vi "getPathPrivate.vi"(1 "bentStyleRef":refnum<class "BentStyle.lvclass">, 2 "start":T2 {"height" format="%.2f"; "width" format="%.2f"; "y" format="%.2f"; "x" format="%.2f"}, 3 "end":T2 {"height" format="%.2f"; "width" format="%.2f"; "y" format="%.2f"; "x" format="%.2f"}, 5 "error in (no error)":errorcluster) -> (15 "path":T3[](array[typedef]) {"y" format="%.2f"; "x" format="%.2f"}, 16 "ok":bool, 17 "startDirection":T1, 18 "endDirection":T1, 19 "error out":errorcluster)   [LabVIEW 2016, in "BentStyle.lvclass"]
doc: "/**\n Gets the points at which a line joining two rectangles\n is bent according to a bent style.\n @param start the starting rectangle\n @param end the ending rectangle\n @return an array list of points at which to bend the\n segmented line joining the two rectangles\n */\n private static ArrayList getPath(BentStyle bent, \n Rectangle2D s, Rectangle2D e)"
uses:
  <resource>/Framework/Providers/Open_GDS/UML/BentStyle_class/BentStyle.lvclass
  <resource>/Framework/Providers/Open_GDS/UML/General/Point/Point Point2D.ctl
  <resource>/Framework/Providers/Open_GDS/UML/General/Rectangle/Rectangle Rectangle2D.ctl
  <resource>/Framework/Providers/Open_GDS/UML/Direction_class/DirectionTypes.ctl
  <resource>/Framework/Providers/Open_GDS/UML/BentStyle_class/BentStyle.lvclass/BentStyle.ctl
  <resource>/Framework/Providers/Open_GDS/UML/Direction_class/Direction.lvclass
panel:
  # "PRIVATE STATIC getPath (BentStyle,Rect,Rect)"
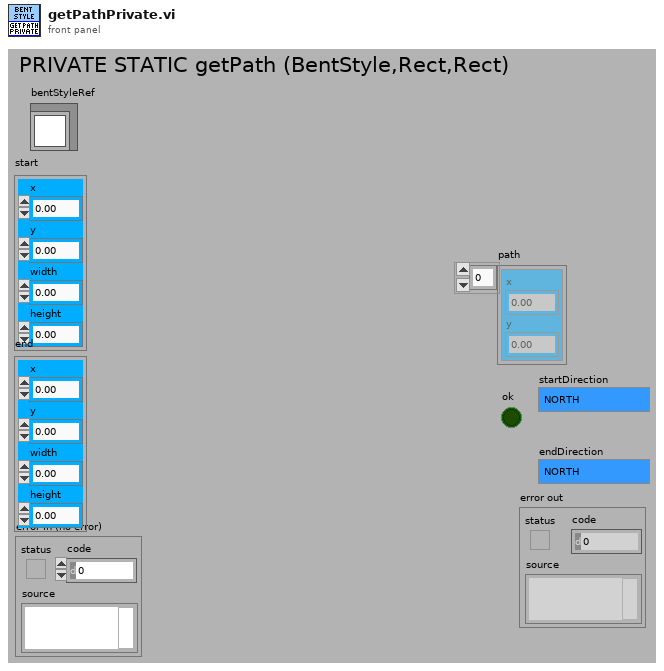
[diagram p1: front panel]
types:
  T1 = typedef "Direction.lvclass/DirectionTypes.ctl" = enum16{"NORTH", "SOUTH", "EAST", "WEST"}
  T2 = typedef "Rectangle Rectangle2D.ctl" = cluster{"x":dbl, "y":dbl, "width":dbl, "height":dbl}
  T3 = typedef "Point Point2D.ctl" = cluster{"x":dbl, "y":dbl}
  T4 = typedef "BentStyle.lvclass/BentStyleType.ctl" = enum16{"STRAIGHT", "HV", "VH", "HVH", "VHV", "ARC"}
  T5 = cluster{"point2D":T3, "point2D":T3, "distance":dbl, i32, i32}
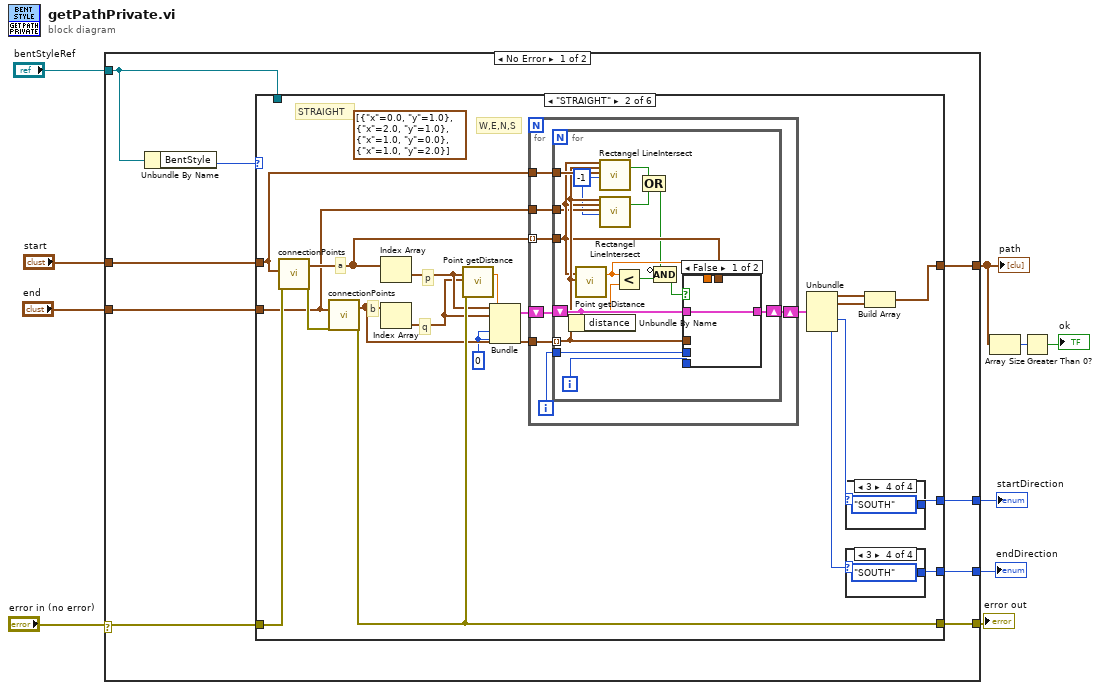
[diagram p0: block diagram]
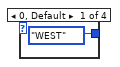
[diagram p3: hidden frame]
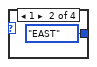
[diagram p4: hidden frame]
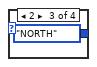
[diagram p5: hidden frame]
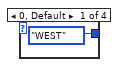
[diagram p6: hidden frame]
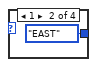
[diagram p7: hidden frame]
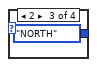
[diagram p8: hidden frame]
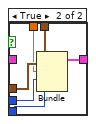
[diagram p9: hidden frame]
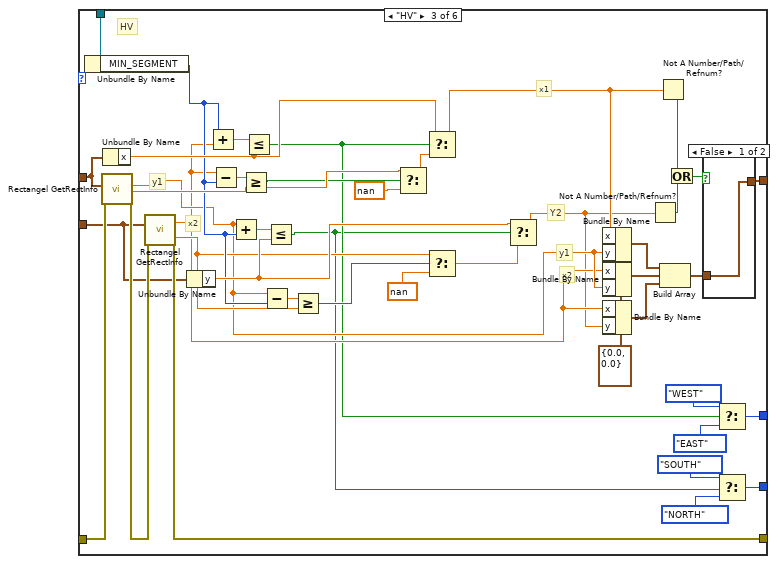
[diagram p10: hidden frame]
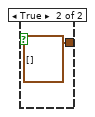
[diagram p11: hidden frame]
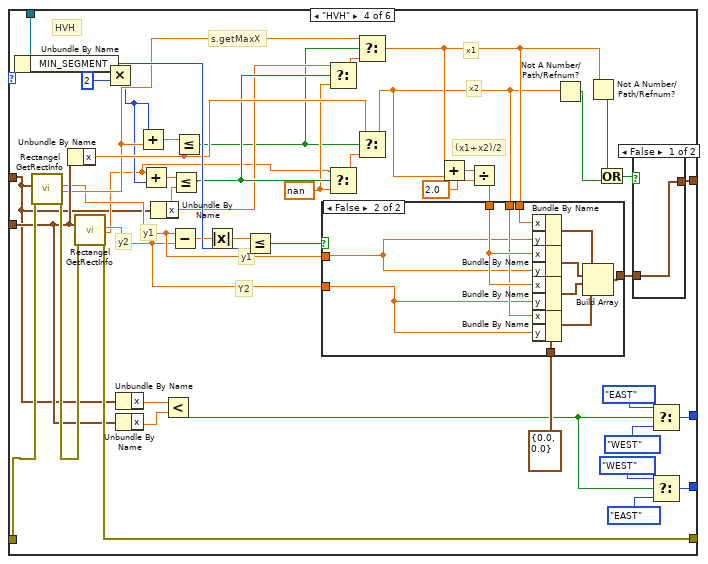
[diagram p12: hidden frame]
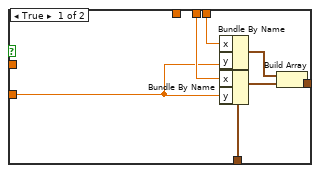
[diagram p13: hidden frame]
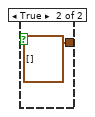
[diagram p14: hidden frame]
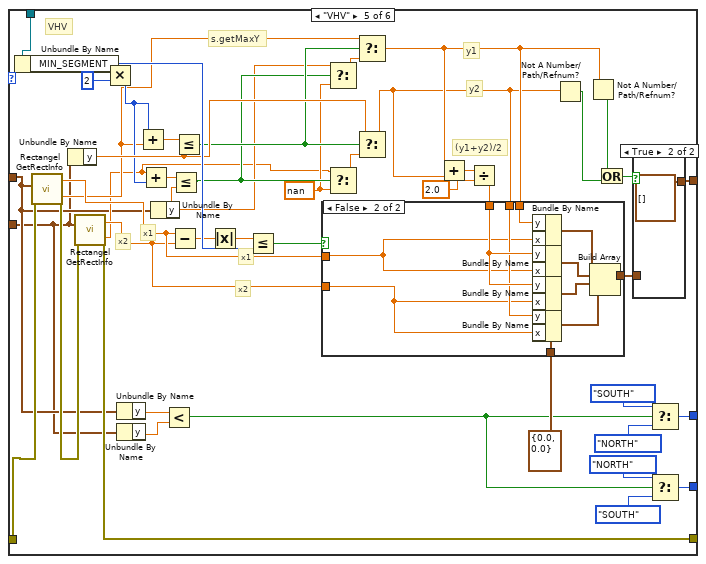
[diagram p15: hidden frame]
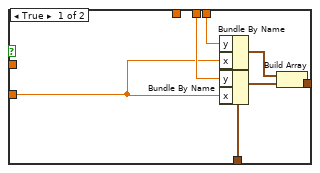
[diagram p16: hidden frame]
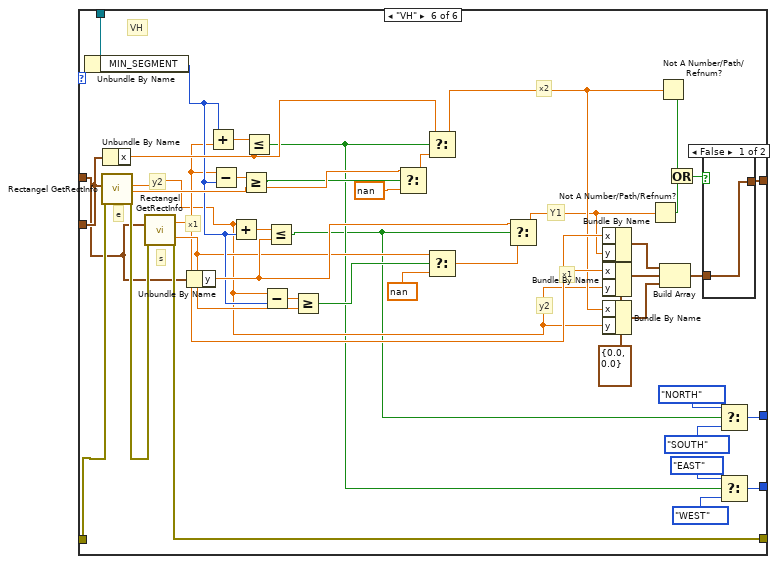
[diagram p18: hidden frame]
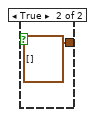
[diagram p19: hidden frame]
diagram:
  n1 = case shown="No Error" "error in (no error)" {
    selector: "error in (no error)" -> [w11 w297]
    tunnel: "bentStyleRef" -> [w13 _]
    tunnel: [w19 w297] -> w9
    tunnel: "start" -> [w18 _]
    tunnel: "end" -> [w17 _]
    tunnel: [w16 _] -> w4
    tunnel: [w15 _] -> w2
    tunnel: [w14 _] -> w1
    frame No Error {
      n2 = Unbundle By Name(w13) -> ("BentStyle"=w12:T4)
      n3 = case shown="\"STRAIGHT\"" w12 {
        tunnel: w11 -> [w20 w24 w119 w166 w231 w293]
        tunnel: [w20 w40 w117 w164 w229 w291] -> w19
        tunnel: w13 -> [_ _ w120 w167 w232 w294]
        tunnel: w18 -> [_ w22 w114 w126 w190 w265]
        tunnel: w17 -> [_ w21 w87 w152 w189 w266]
        tunnel: [_ w31 w116 w163 w228 w290] -> w16
        tunnel: [_ w27 w86 w129 w194 w256] -> w15
        tunnel: [_ w26 w81 w128 w193 w255] -> w14
        frame Default {
          # "Default"
        }
        frame "STRAIGHT" {
          (unwired) T3[] [{"x"=0.0, "y"=1.0}, {"x"=2.0, "y"=1.0}, {"x"=1.0, "y"=0.0}, {"x"=1.0, "y"=2.0}] ("path")
          w29 = 0
          # "STRAIGHT"
          # "W,E,N,S"
          # "q"
          # "p"
          # "b"
          # "a"
          n4 = call <resource>:"connectionPoints.vi"("r"=w22, "error in (no error)"=w24) -> ("path"=w39:T3[], "error out"=w23:errorcluster)  [unwired: 16 out]
          n5 = call <resource>:"connectionPoints.vi"("r"=w21, "error in (no error)"=w23) -> ("path"=w38:T3[], "error out"=w40:errorcluster)  [unwired: 16 out]
          n6 = Index Array(array=w39) -> (element=w37:T3)  [unwired: 1 in]
          n7 = Index Array(array=w38) -> (element=w36:T3)  [unwired: 1 in]
          n8 = call <resource>:"Point getDistance.vi"("point1"=w37, "point2"=w36, "error in (no error)"=w40) -> ("distance"=w30:dbl)  [unwired: 16 out]
          n9 = Bundle("point2D"=w37, "point2D"=w36, "distance"=w30, w29, w29) -> (w35:T5)  [unwired: 1 out]
          n10 = for {
            tunnel: w39 -> [w52] mode=indexing
            tunnel: w38 -> [w55]
            shift-right: [w53] -> w34
            shift-left: w35 -> [w54]
            tunnel: w22 -> [w50]
            tunnel: w21 -> [w49]
            i -> [w51]
            n11 = for {
              tunnel: w55 -> [w64] mode=indexing
              shift-right: [w71] -> w53
              shift-left: w54 -> [w70]
              tunnel: w52 -> [w63]
              tunnel: w51 -> [w67]
              tunnel: w50 -> [w65]
              tunnel: w49 -> [w62]
              i -> [w66]
              w56 = -1 ("Margin")
              n12 = Unbundle By Name(w70) -> ("distance"=w69:dbl)
              n13 = call <resource>:"Point getDistance.vi"("point1"=w63, "point2"=w64) -> ("distance"=w68:dbl)  [unwired: 1 in, 16 out]
              n14 = call <resource>:"Rectangel LineIntersect.vi"("LinePoint1"=w63, "LinePoint2"=w64, "bounds"=w65, "Margin"=w56) -> ("Intersect"=w59:bool)  [unwired: 14 in, 1 out]
              n15 = call <resource>:"Rectangel LineIntersect.vi"("LinePoint1"=w64, "LinePoint2"=w63, "bounds"=w62, "Margin"=w56) -> ("Intersect"=w58:bool)  [unwired: 14 in, 1 out]
              n16 = Less?(x=w68, y=w69) -> (x < y?=w61:bool)
              n17 = Compound Arithmetic op=OR(w59, w58) -> (w57:bool)
              n18 = Compound Arithmetic op=AND(invert w57, w61) -> (w60:bool)
              n19 = case shown="False" w60 {
                tunnel: w70 -> [w72 _]
                tunnel: [w72 w78] -> w71
                tunnel: w63 -> [_ w77]
                tunnel: w64 -> [_ w76]
                tunnel: w68 -> [_ w75]
                tunnel: w67 -> [_ w74]
                tunnel: w66 -> [_ w73]
                frame False {
                }
                frame True {
                  n20 = Bundle("point2D"=w77, "point2D"=w76, "distance"=w75, w74, w73) -> (w78:T5)  [unwired: 1 out]
                }
              }
            }
          }
          n21 = Unbundle(w34) -> ("point2D"=w33:T3, "point2D"=w32:T3, w28:i32, w25:i32)  [unwired: 1 out]
          n22 = case shown="3" w28 {
            tunnel: [DirectionTypes."WEST" ("startDirection") DirectionTypes."EAST" ("startDirection") DirectionTypes."NORTH" ("startDirection") DirectionTypes."SOUTH" ("startDirection")] -> w27
            frame 0, Default {
            }
            frame 1 {
            }
            frame 2 {
            }
            frame 3 {
            }
          }
          n23 = case shown="3" w25 {
            tunnel: [DirectionTypes."WEST" ("startDirection") DirectionTypes."EAST" ("startDirection") DirectionTypes."NORTH" ("startDirection") DirectionTypes."SOUTH" ("startDirection")] -> w26
            frame 0, Default {
            }
            frame 1 {
            }
            frame 2 {
            }
            frame 3 {
            }
          }
          n24 = Build Array(w33, w32) -> (w31:T3[])
        }
        frame "HV" {
          w95 = T3 {"x"=0.0, "y"=0.0} ("point2D")
          # "HV"
          # "x2"
          # "y1"
          # "Y2"
          # "x1"
          # "x2"
          # "y1"
          n25 = Unbundle By Name(w120) -> ("MIN_SEGMENT"=w105:i32)
          n26 = call <resource>:"Rectangel GetRectInfo.vi"("bounds"=w114, "error in (no error)"=w119) -> ("centerY"=w90:dbl, "maxX"=w111:dbl, "error out"=w118:errorcluster)  [unwired: 15 out]
          n27 = Unbundle By Name(w114) -> ("x"=w113:dbl)
          n28 = call <resource>:"Rectangel GetRectInfo.vi"("bounds"=w87, "error in (no error)"=w118) -> ("centerX"=w89:dbl, "maxY"=w103:dbl, "error out"=w117:errorcluster)  [unwired: 15 out]
          n29 = Unbundle By Name(w87) -> ("y"=w106:dbl)
          n30 = Add(x=w105, y=w89) -> (x+y=w115:dbl)
          n31 = Subtract(x=w89, y=w105) -> (x-y=w112:dbl)
          n32 = Add(x=w90, y=w105) -> (x+y=w107:dbl)
          n33 = Greater Or Equal?(x=w112, y=w111) -> (x >= y?=w110:bool)
          n34 = Less Or Equal?(x=w115, y=w113) -> (x <= y?=w80:bool)
          n35 = Subtract(x=w90, y=w105) -> (x-y=w104:dbl)
          n36 = Less Or Equal?(x=w107, y=w106) -> (x <= y?=w79:bool)
          n37 = Greater Or Equal?(x=w104, y=w103) -> (x >= y?=w102:bool)
          n38 = Select(t=w111, s=w110, f=nan) -> (s? t:f=w109:dbl)
          n39 = Select(t=w113, s=w80, f=w109) -> (s? t:f=w91:dbl)
          n40 = Select(t=w103, s=w102, f=nan) -> (s? t:f=w100:dbl)
          n41 = Select(t=w106, s=w79, f=w100) -> (s? t:f=w88:dbl)
          n42 = Bundle By Name(cluster=w95, "x"=w91, "y"=w90) -> (w92:T3)
          n43 = Bundle By Name(cluster=w95, "x"=w89, "y"=w90) -> (w94:T3)
          n44 = Bundle By Name(cluster=w95, "x"=w89, "y"=w88) -> (w93:T3)
          n45 = Not A Number/Path/Refnum?(number/path/refnum=w88) -> (NaN/Path/Refnum?=w98:bool)
          n46 = Not A Number/Path/Refnum?(number/path/refnum=w91) -> (NaN/Path/Refnum?=w99:bool)
          n47 = Build Array(w92, w94, w93) -> (w96:T3[])
          n48 = Or(x=w99, y=w98) -> (x .or. y?=w97:bool)
          n49 = case shown="False" w97 {
            tunnel: [w121 T3[] [] ("path")] -> w116
            tunnel: w96 -> [w121 _]
            frame False {
            }
            frame True {
            }
          }
          n50 = Select(t=DirectionTypes."WEST" ("startDirection"), s=w80, f=DirectionTypes."EAST" ("startDirection")) -> (s? t:f=w86:T1)
          n51 = Select(t=DirectionTypes."SOUTH" ("startDirection"), s=w79, f=DirectionTypes."NORTH" ("startDirection")) -> (s? t:f=w81:T1)
        }
        frame "HVH" {
          w148 = nan ("f")
          # "HVH"
          # "(x1+x2)/2"
          # "y1"
          # "s.getMaxX"
          # "x1"
          # "Y2"
          # "x2"
          # "y2"
          # "y1"
          n52 = Unbundle By Name(w167) -> ("MIN_SEGMENT"=w159:i32)
          n53 = call <resource>:"Rectangel GetRectInfo.vi"("bounds"=w126, "error in (no error)"=w166) -> ("centerY"=w142:dbl, "maxX"=w150:dbl, "error out"=w165:errorcluster)  [unwired: 15 out]
          n54 = Unbundle By Name(w152) -> ("x"=w151:dbl)
          n55 = call <resource>:"Rectangel GetRectInfo.vi"("bounds"=w152, "error in (no error)"=w165) -> ("centerY"=w141:dbl, "maxX"=w134:dbl, "error out"=w164:errorcluster)  [unwired: 15 out]
          n56 = Multiply(x=w159, y=2) -> (x*y=w145:i32)
          n57 = Unbundle By Name(w126) -> ("x"=w125:dbl)
          n58 = Unbundle By Name(w152) -> ("x"=w124:dbl)
          n59 = Add(x=w145, y=w150) -> (x+y=w162:dbl)
          n60 = Add(x=w134, y=w145) -> (x+y=w161:dbl)
          n61 = Unbundle By Name(w126) -> ("x"=w146:dbl)
          n62 = Less?(x=w125, y=w124) -> (x < y?=w123:bool)
          n63 = Subtract(x=w142, y=w141) -> (x-y=w144:dbl)
          n64 = Less Or Equal?(x=w161, y=w146) -> (x <= y?=w149:bool)
          n65 = Less Or Equal?(x=w162, y=w151) -> (x <= y?=w127:bool)
          n66 = Absolute Value(x=w144) -> (abs(x)=w135:dbl)
          n67 = Less Or Equal?(x=w135, y=w159) -> (x <= y?=w143:bool)
          n68 = Select(t=w146, s=w149, f=w148) -> (s? t:f=w147:dbl)
          n69 = Select(t=w134, s=w149, f=w148) -> (s? t:f=w160:dbl)
          n70 = Select(t=w150, s=w127, f=w147) -> (s? t:f=w140:dbl)
          n71 = Select(t=w151, s=w127, f=w160) -> (s? t:f=w139:dbl)
          n72 = Add(x=w140, y=w139) -> (x+y=w138:dbl)
          n73 = Divide(x=w138, y=2.0) -> (x/y=w136:dbl)
          n74 = case shown="False" w143 {
            tunnel: [w174 w185] -> w155
            tunnel: T3 {"x"=0.0, "y"=0.0} ("point2D") -> [w173 w181]
            tunnel: w140 -> [w170 w179]
            tunnel: w139 -> [w169 w177]
            tunnel: w142 -> [_ w176]
            tunnel: w141 -> [w168 w175]
            tunnel: w136 -> [_ w178]
            frame True {
              n75 = Bundle By Name(cluster=w173, "x"=w170, "y"=w168) -> (w171:T3)
              n76 = Bundle By Name(cluster=w173, "x"=w169, "y"=w168) -> (w172:T3)
              n77 = Build Array(w171, w172) -> (w174:T3[])
            }
            frame False {
              n78 = Bundle By Name(cluster=w181, "x"=w179, "y"=w176) -> (w182:T3)
              n79 = Bundle By Name(cluster=w181, "x"=w178, "y"=w176) -> (w184:T3)
              n80 = Bundle By Name(cluster=w181, "x"=w178, "y"=w175) -> (w183:T3)
              n81 = Bundle By Name(cluster=w181, "x"=w177, "y"=w175) -> (w180:T3)
              n82 = Build Array(w182, w184, w183, w180) -> (w185:T3[])
            }
          }
          n83 = Not A Number/Path/Refnum?(number/path/refnum=w139) -> (NaN/Path/Refnum?=w157:bool)
          n84 = Not A Number/Path/Refnum?(number/path/refnum=w140) -> (NaN/Path/Refnum?=w158:bool)
          n85 = Or(x=w158, y=w157) -> (x .or. y?=w156:bool)
          n86 = case shown="False" w156 {
            tunnel: [w186 T3[] [] ("path")] -> w163
            tunnel: w155 -> [w186 _]
            frame False {
            }
            frame True {
            }
          }
          n87 = Select(t=DirectionTypes."EAST" ("startDirection"), s=w123, f=DirectionTypes."WEST" ("startDirection")) -> (s? t:f=w129:T1)
          n88 = Select(t=DirectionTypes."WEST" ("startDirection"), s=w123, f=DirectionTypes."EAST" ("startDirection")) -> (s? t:f=w128:T1)
        }
        frame "VHV" {
          w214 = nan ("f")
          # "VHV"
          # "(y1+y2)/2"
          # "x1"
          # "s.getMaxY"
          # "y1"
          # "x2"
          # "y2"
          # "x2"
          # "x1"
          n89 = Unbundle By Name(w232) -> ("MIN_SEGMENT"=w224:i32)
          n90 = call <resource>:"Rectangel GetRectInfo.vi"("bounds"=w190, "error in (no error)"=w231) -> ("centerX"=w203:dbl, "maxY"=w201:dbl, "error out"=w230:errorcluster)  [unwired: 15 out]
          n91 = Unbundle By Name(w189) -> ("y"=w217:dbl)
          n92 = call <resource>:"Rectangel GetRectInfo.vi"("bounds"=w189, "error in (no error)"=w230) -> ("centerX"=w202:dbl, "maxY"=w200:dbl, "error out"=w229:errorcluster)  [unwired: 15 out]
          n93 = Multiply(x=w224, y=2) -> (x*y=w211:i32)
          n94 = Unbundle By Name(w190) -> ("y"=w192:dbl)
          n95 = Unbundle By Name(w189) -> ("y"=w191:dbl)
          n96 = Add(x=w211, y=w201) -> (x+y=w227:dbl)
          n97 = Add(x=w200, y=w211) -> (x+y=w226:dbl)
          n98 = Unbundle By Name(w190) -> ("y"=w212:dbl)
          n99 = Less?(x=w192, y=w191) -> (x < y?=w188:bool)
          n100 = Subtract(x=w203, y=w202) -> (x-y=w210:dbl)
          n101 = Less Or Equal?(x=w226, y=w212) -> (x <= y?=w215:bool)
          n102 = Less Or Equal?(x=w227, y=w217) -> (x <= y?=w216:bool)
          n103 = Absolute Value(x=w210) -> (abs(x)=w199:dbl)
          n104 = Less Or Equal?(x=w199, y=w224) -> (x <= y?=w209:bool)
          n105 = Select(t=w212, s=w215, f=w214) -> (s? t:f=w213:dbl)
          n106 = Select(t=w200, s=w215, f=w214) -> (s? t:f=w225:dbl)
          n107 = Select(t=w201, s=w216, f=w213) -> (s? t:f=w208:dbl)
          n108 = Select(t=w217, s=w216, f=w225) -> (s? t:f=w207:dbl)
          n109 = Add(x=w208, y=w207) -> (x+y=w206:dbl)
          n110 = Divide(x=w206, y=2.0) -> (x/y=w204:dbl)
          n111 = case shown="False" w209 {
            tunnel: [w239 w250] -> w220
            tunnel: T3 {"x"=0.0, "y"=0.0} ("point2D") -> [w238 w246]
            tunnel: w208 -> [w235 w244]
            tunnel: w207 -> [w234 w242]
            tunnel: w203 -> [_ w241]
            tunnel: w202 -> [w233 w240]
            tunnel: w204 -> [_ w243]
            frame True {
              n112 = Bundle By Name(cluster=w238, "y"=w235, "x"=w233) -> (w236:T3)
              n113 = Bundle By Name(cluster=w238, "y"=w234, "x"=w233) -> (w237:T3)
              n114 = Build Array(w236, w237) -> (w239:T3[])
            }
            frame False {
              n115 = Bundle By Name(cluster=w246, "y"=w244, "x"=w241) -> (w247:T3)
              n116 = Bundle By Name(cluster=w246, "y"=w243, "x"=w241) -> (w249:T3)
              n117 = Bundle By Name(cluster=w246, "y"=w243, "x"=w240) -> (w248:T3)
              n118 = Bundle By Name(cluster=w246, "y"=w242, "x"=w240) -> (w245:T3)
              n119 = Build Array(w247, w249, w248, w245) -> (w250:T3[])
            }
          }
          n120 = Not A Number/Path/Refnum?(number/path/refnum=w207) -> (NaN/Path/Refnum?=w222:bool)
          n121 = Not A Number/Path/Refnum?(number/path/refnum=w208) -> (NaN/Path/Refnum?=w223:bool)
          n122 = Or(x=w223, y=w222) -> (x .or. y?=w221:bool)
          n123 = case shown="True" w221 {
            tunnel: [w251 T3[] [] ("path")] -> w228
            tunnel: w220 -> [w251 _]
            frame False {
            }
            frame True {
            }
          }
          n124 = Select(t=DirectionTypes."SOUTH" ("startDirection"), s=w188, f=DirectionTypes."NORTH" ("startDirection")) -> (s? t:f=w194:T1)
          n125 = Select(t=DirectionTypes."NORTH" ("startDirection"), s=w188, f=DirectionTypes."SOUTH" ("startDirection")) -> (s? t:f=w193:T1)
        }
        frame "VH" {
          w270 = T3 {"x"=0.0, "y"=0.0} ("point2D")
          # "VH"
          # "e"
          # "s"
          # "x1"
          # "y2"
          # "Y1"
          # "x2"
          # "x1"
          # "y2"
          n126 = Unbundle By Name(w294) -> ("MIN_SEGMENT"=w280:i32)
          n127 = call <resource>:"Rectangel GetRectInfo.vi"("bounds"=w266, "error in (no error)"=w293) -> ("centerY"=w261:dbl, "maxX"=w286:dbl, "error out"=w292:errorcluster)  [unwired: 15 out]
          n128 = Unbundle By Name(w266) -> ("x"=w288:dbl)
          n129 = call <resource>:"Rectangel GetRectInfo.vi"("bounds"=w265, "error in (no error)"=w292) -> ("centerX"=w264:dbl, "maxY"=w278:dbl, "error out"=w291:errorcluster)  [unwired: 15 out]
          n130 = Unbundle By Name(w265) -> ("y"=w281:dbl)
          n131 = Add(x=w280, y=w264) -> (x+y=w289:dbl)
          n132 = Subtract(x=w264, y=w280) -> (x-y=w287:dbl)
          n133 = Add(x=w261, y=w280) -> (x+y=w282:dbl)
          n134 = Greater Or Equal?(x=w287, y=w286) -> (x >= y?=w285:bool)
          n135 = Less Or Equal?(x=w289, y=w288) -> (x <= y?=w254:bool)
          n136 = Subtract(x=w261, y=w280) -> (x-y=w279:dbl)
          n137 = Less Or Equal?(x=w282, y=w281) -> (x <= y?=w253:bool)
          n138 = Greater Or Equal?(x=w279, y=w278) -> (x >= y?=w277:bool)
          n139 = Select(t=w286, s=w285, f=nan) -> (s? t:f=w284:dbl)
          n140 = Select(t=w288, s=w254, f=w284) -> (s? t:f=w263:dbl)
          n141 = Select(t=w278, s=w277, f=nan) -> (s? t:f=w275:dbl)
          n142 = Select(t=w281, s=w253, f=w275) -> (s? t:f=w262:dbl)
          n143 = Bundle By Name(cluster=w270, "x"=w264, "y"=w262) -> (w267:T3)
          n144 = Bundle By Name(cluster=w270, "x"=w264, "y"=w261) -> (w269:T3)
          n145 = Bundle By Name(cluster=w270, "x"=w263, "y"=w261) -> (w268:T3)
          n146 = Not A Number/Path/Refnum?(number/path/refnum=w262) -> (NaN/Path/Refnum?=w273:bool)
          n147 = Not A Number/Path/Refnum?(number/path/refnum=w263) -> (NaN/Path/Refnum?=w274:bool)
          n148 = Build Array(w267, w269, w268) -> (w271:T3[])
          n149 = Or(x=w274, y=w273) -> (x .or. y?=w272:bool)
          n150 = case shown="False" w272 {
            tunnel: [w295 T3[] [] ("path")] -> w290
            tunnel: w271 -> [w295 _]
            frame False {
            }
            frame True {
            }
          }
          n151 = Select(t=DirectionTypes."NORTH" ("startDirection"), s=w253, f=DirectionTypes."SOUTH" ("startDirection")) -> (s? t:f=w256:T1)
          n152 = Select(t=DirectionTypes."EAST" ("startDirection"), s=w254, f=DirectionTypes."WEST" ("startDirection")) -> (s? t:f=w255:T1)
        }
      }
    }
    frame Error {
    }
  }
  "error out" <- w9
  "path" <- w4
  "startDirection" <- w2
  "endDirection" <- w1
  n153 = Array Size(array=w4) -> (size(s)=w5:i32)
  n154 = Greater Than 0?(x=w5) -> (x > 0?=→"ok":bool)
